vi "OSC_Calc-1.vi"(8 "Flow":dbl, 9 "Lambda 2 Array":dbl[](array[numeric]), 10 "Lambda 1 Array":dbl[](array[numeric]), 11 "MFC":dbl) -> (1 "OSC-Meas Flow":dbl, 2 "OSC- Calc Flow":dbl, 3 "Calculated Flow":dbl)   [LabVIEW 2014]
uses:
  <vilib>/Analysis/baseanly.llb/Mean (DBL).vi
  <vilib>/Analysis/NI_AALPro.lvlib
  <vilib>/Analysis/NI_AALBase.lvlib
panel:
  out "After TP 1":i32
  out "After TP 2":i32
  out "Time":dbl
  out "mean":dbl format="%0.2f"
  out "mean 2":dbl format="%0.2f"
  out "mean 3":dbl format="%0.2f"
  out "L1 Gradient":dbl[](graph)
  out "L1 Avg Gradient":dbl[](graph)
  out "L1 Data":dbl[](graph)
  out "L1 Max Grad":dbl
  out "L1 TP":i32
  out "L2 Gradient":dbl[](graph)
  out "L2 Avg Gradient":dbl[](graph)
  out "L2 Data":dbl[](graph)
  out "L2 Max Grad":dbl
  out "L2 TP":i32
  # "OSC Calculation"
  # "Inputs"
  # "Outputs"
  # "Indicators"
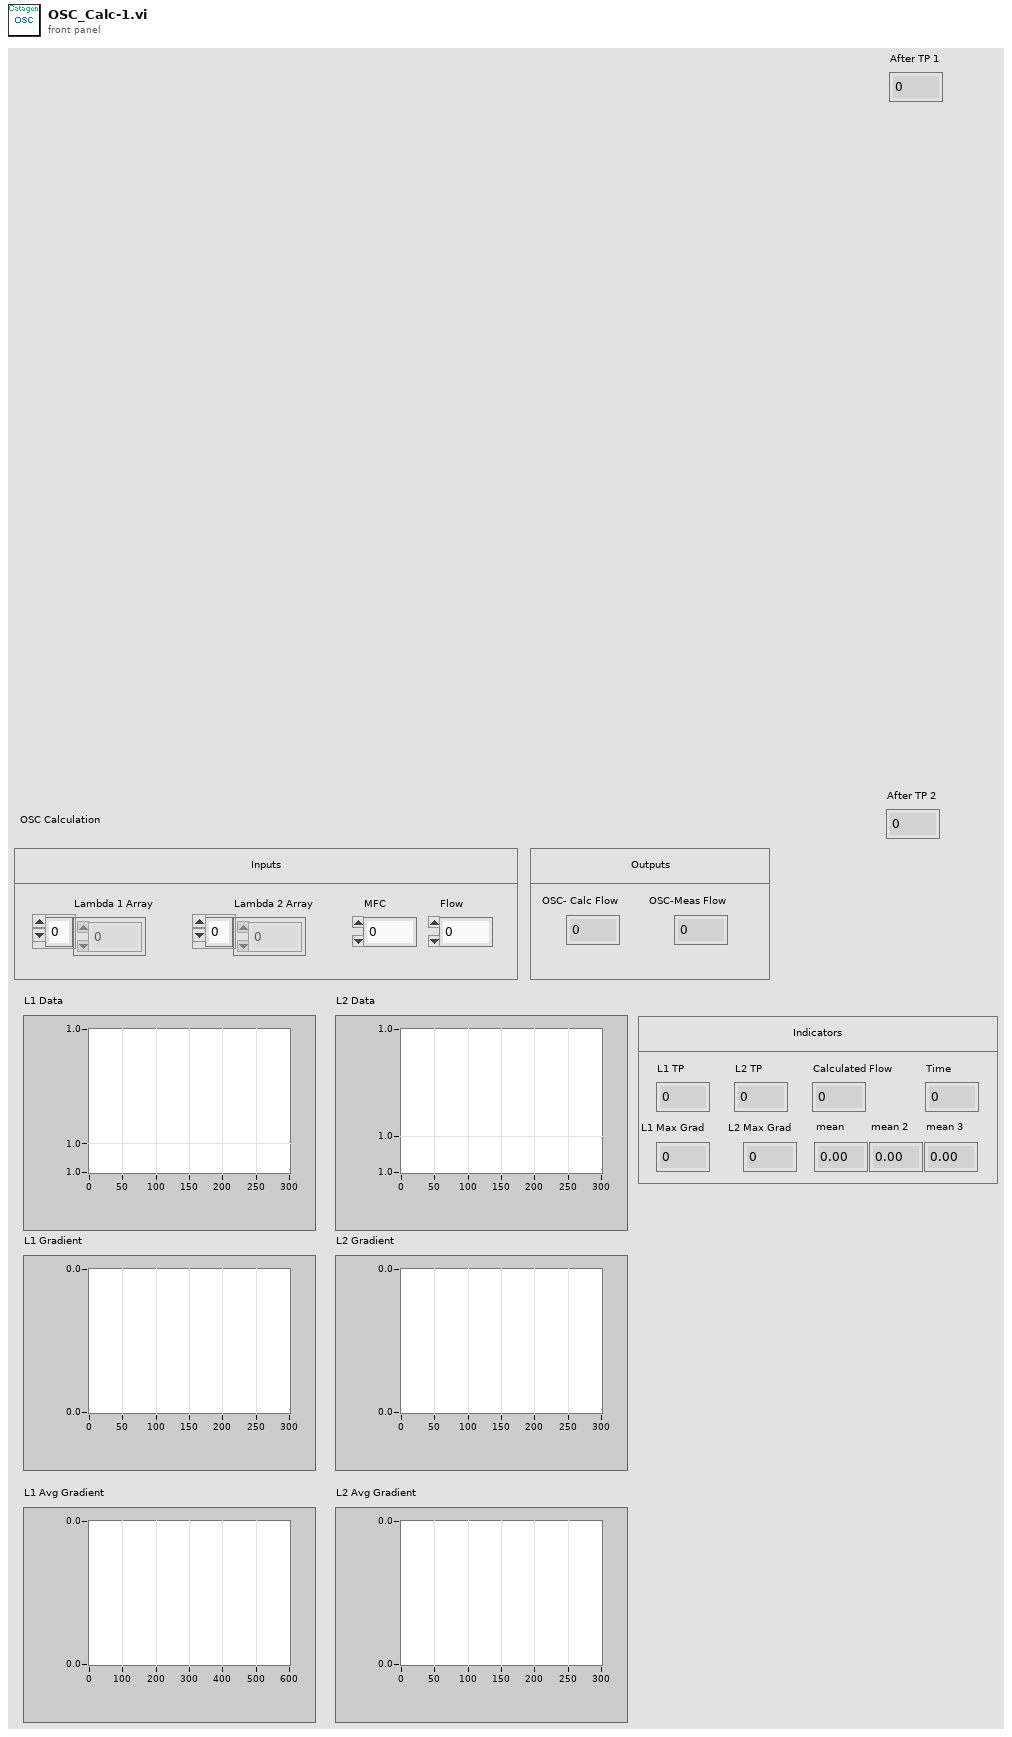
[diagram p1: front panel]
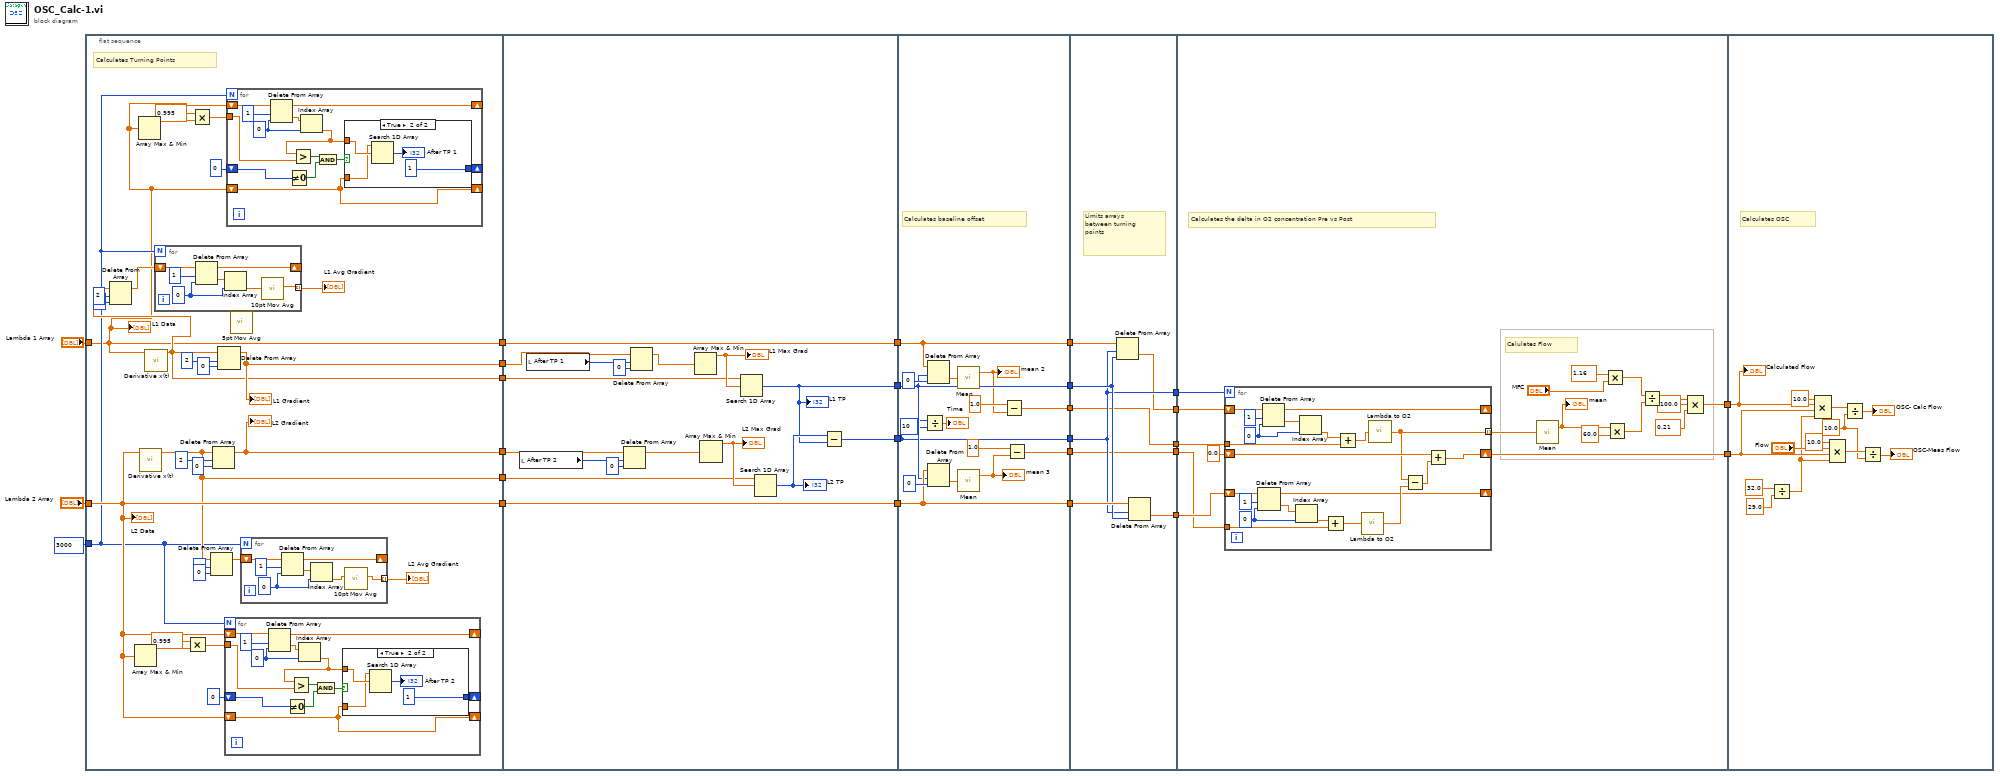
[diagram p0: block diagram]
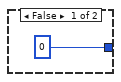
[diagram p2: hidden frame]
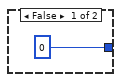
[diagram p3: hidden frame]
diagram:
  n1 = flat-sequence {
    tunnel: [w37] -> w10
    tunnel: [w27] -> w8
    tunnel: "Lambda 1 Array" -> [w27]
    tunnel: "Lambda 2 Array" -> [w37]
    tunnel: 3000 -> [w32]
    tunnel: [w36] -> w4
    tunnel: [w35] -> w3
    tunnel: [w34] -> w2
    tunnel: [w33] -> w1
    tunnel: w10 -> [w120]
    tunnel: [w120] -> w9
    tunnel: w8 -> [w119]
    tunnel: [w119] -> w7
    tunnel: [w115] -> w6
    tunnel: [w104] -> w5
    tunnel: w4 -> [w105]
    tunnel: w3 -> [w114]
    tunnel: w2 -> [w113]
    tunnel: w1 -> [w112]
    tunnel: w9 -> [w131]
    tunnel: [w131] -> w26
    tunnel: w7 -> [w136]
    tunnel: [w136] -> w25
    tunnel: w6 -> [w123]
    tunnel: [w123] -> w24
    tunnel: w5 -> [w130]
    tunnel: [w130] -> w23
    tunnel: [w128] -> w22
    tunnel: [w124] -> w12
    tunnel: w26 -> [w143]
    tunnel: w25 -> [w144]
    tunnel: w24 -> [w141]
    tunnel: w23 -> [w142]
    tunnel: [w141] -> w21
    tunnel: [w140] -> w20
    tunnel: [w139] -> w19
    tunnel: w22 -> [w138]
    tunnel: [w138] -> w18
    tunnel: w12 -> [w137]
    tunnel: [w137] -> w11
    tunnel: w21 -> [w162]
    tunnel: w20 -> [w160]
    tunnel: w19 -> [w161]
    tunnel: [w158] -> w17
    tunnel: [w147] -> w16
    tunnel: w18 -> [w146]
    tunnel: w11 -> [w145]
    tunnel: w17 -> [w191]
    tunnel: w16 -> [w195]
    frame #0 {
      # "Calculates Turning Points"
      n2 = Array Max & Min(array=w37) -> (max value=w41:dbl)  [unwired: 3 out]
      n3 = Array Max & Min(array=w27) -> (max value=w30:dbl)  [unwired: 3 out]
      n4 = call <vilib>:"Derivative x(t).vi"("X"=w37) -> ("dX/dt"=w34:dbl[])  [unwired: 9 in, 1 out]
      n5 = call <vilib>:"Derivative x(t).vi"("X"=w27) -> ("dX/dt"=w35:dbl[])  [unwired: 9 in, 1 out]
      n6 = Delete From Array(array=w35, length=2, index=0) -> (array with subset deleted=w44:dbl[])  [unwired: 1 out]
      n7 = for {
        N: w32 -> [_]
        tunnel: [w97] -> w48 mode=indexing
        shift-right: [w102] -> _
        shift-left: w44 -> [w101]
        w99 = 0 ("index")
        n8 = Delete From Array(array=w101, length=1, index=w99) -> (deleted portion=w100:dbl[], array with subset deleted=w102:dbl[])
        n9 = Index Array(array=w100, index=w99) -> (element=w98:dbl)
        n10 = call "10pt Mov Avg.vi"("Value in"=w98) -> ("Value out"=w97:dbl)  [unwired: 10 in]
      }
      "L1 Avg Gradient" <- w48
      n11 = Multiply(x=0.995, y=w41) -> (x*y=w39:dbl)
      n12 = Multiply(x=0.995, y=w30) -> (x*y=w29:dbl)
      n13 = Delete From Array(array=w34, length=2, index=0) -> (array with subset deleted=w45:dbl[])  [unwired: 1 out]
      n14 = Delete From Array(array=w34, length=2, index=0) -> (array with subset deleted=w33:dbl[])  [unwired: 1 out]
      "L2 Gradient" <- w33
      n15 = Delete From Array(array=w35, length=2, index=0) -> (array with subset deleted=w36:dbl[])  [unwired: 1 out]
      "L1 Gradient" <- w36
      n16 = for {
        N: w32 -> [_]
        tunnel: w39 -> [w77]
        shift-right: [w84] -> _
        shift-left: w37 -> [w83]
        shift-right: [w74] -> _
        shift-left: 0 ("index") -> [w73]
        shift-right: [w72] -> _
        shift-left: w37 -> [w72]
        w81 = 0 ("index")
        n17 = Delete From Array(array=w83, length=1, index=w81) -> (deleted portion=w82:dbl[], array with subset deleted=w84:dbl[])
        n18 = Not Equal To 0?(x=w73) -> (x != 0?=w75:bool)
        n19 = Index Array(array=w82, index=w81) -> (element=w76:dbl)
        n20 = Greater?(x=w76, y=w77) -> (0:w78:bool)
        n21 = And(x=w78, y=w75) -> (x .and. y?=w79:bool)
        n22 = case shown="True" w79 {
          tunnel: w76 -> [_ w88]
          tunnel: [0 ("index") 1 ("index")] -> w74
          tunnel: w72 -> [_ w87]
          frame False {
          }
          frame True {
            n23 = Search 1D Array(1D array=w87, element=w88) -> (index of element=→"After TP 2":i32)  [unwired: 1 in]
          }
        }
      }
      n24 = for {
        N: w32 -> [_]
        tunnel: w29 -> [w59]
        shift-right: [w66] -> _
        shift-left: w27 -> [w65]
        shift-right: [w56] -> _
        shift-left: 0 ("index") -> [w55]
        shift-right: [w54] -> _
        shift-left: w27 -> [w54]
        w63 = 0 ("index")
        n25 = Delete From Array(array=w65, length=1, index=w63) -> (deleted portion=w64:dbl[], array with subset deleted=w66:dbl[])
        n26 = Not Equal To 0?(x=w55) -> (x != 0?=w57:bool)
        n27 = Index Array(array=w64, index=w63) -> (element=w58:dbl)
        n28 = Greater?(x=w58, y=w59) -> (0:w60:bool)
        n29 = And(x=w60, y=w57) -> (x .and. y?=w61:bool)
        n30 = case shown="True" w61 {
          tunnel: w58 -> [_ w70]
          tunnel: [0 ("index") 1 ("index")] -> w56
          tunnel: w54 -> [_ w69]
          frame False {
          }
          frame True {
            n31 = Search 1D Array(1D array=w69, element=w70) -> (index of element=→"After TP 1":i32)  [unwired: 1 in]
          }
        }
      }
      n32 = call "5pt Mov Avg.vi"() -> ()  [unwired: 11 in, 1 out]
      n33 = for {
        N: w32 -> [_]
        tunnel: [w90] -> w49 mode=indexing
        shift-right: [w95] -> _
        shift-left: w45 -> [w94]
        w92 = 0 ("index")
        n34 = Delete From Array(array=w94, length=1, index=w92) -> (deleted portion=w93:dbl[], array with subset deleted=w95:dbl[])
        n35 = Index Array(array=w93, index=w92) -> (element=w91:dbl)
        n36 = call "10pt Mov Avg.vi"("Value in"=w91) -> ("Value out"=w90:dbl)  [unwired: 10 in]
      }
      "L2 Avg Gradient" <- w49
      "L1 Data" <- w27
      "L2 Data" <- w37
    }
    frame #1 {
      n37 = local read "After TP 2"() -> (w109:i32)
      n38 = local read "After TP 1"() -> (w108:i32)
      n39 = Delete From Array(array=w112, length=w109, index=0) -> (array with subset deleted=w111:dbl[])  [unwired: 1 out]
      n40 = Delete From Array(array=w105, length=w108, index=0) -> (array with subset deleted=w106:dbl[])  [unwired: 1 out]
      n41 = Array Max & Min(array=w106) -> (max value=w116:dbl)  [unwired: 3 out]
      "L1 Max Grad" <- w116
      n42 = Array Max & Min(array=w111) -> (max value=w117:dbl)  [unwired: 3 out]
      "L2 Max Grad" <- w117
      n43 = Search 1D Array(1D array=w114, element=w116) -> (index of element=w104:i32)  [unwired: 1 in]
      "L1 TP" <- w104
      n44 = Search 1D Array(1D array=w113, element=w117) -> (index of element=w118:i32)  [unwired: 1 in]
      "L2 TP" <- w118
      n45 = Subtract(x=w118, y=w104) -> (x-y=w115:i32)
    }
    frame #2 {
      # "Calculates baseline offset"
      n46 = Divide(x=w123, y=10) -> (x/y=→"Time":dbl)
      n47 = Delete From Array(array=w136, length=w130, index=0) -> (deleted portion=w134:dbl[])  [unwired: 1 out]
      n48 = Delete From Array(array=w131, length=w130, index=0) -> (deleted portion=w133:dbl[])  [unwired: 1 out]
      n49 = call-poly <vilib>:"Mean.vi"("X"=w134) -> ("mean"=w126:dbl)  [unwired: 1 out]
      "mean 2" <- w126
      n50 = call-poly <vilib>:"Mean.vi"("X"=w133) -> ("mean"=w129:dbl)  [unwired: 1 out]
      "mean 3" <- w129
      n51 = Subtract(x=1.0, y=w126) -> (x-y=w124:dbl)
      n52 = Subtract(x=1.0, y=w129) -> (x-y=w128:dbl)
    }
    frame #3 {
      # "Limits arrays\nbetween turning\npoints"
      n53 = Delete From Array(array=w144, length=w141, index=w142) -> (deleted portion=w139:dbl[])  [unwired: 1 out]
      n54 = Delete From Array(array=w143, length=w141, index=w142) -> (deleted portion=w140:dbl[])  [unwired: 1 out]
    }
    frame #4 {
      # "Calculates the delta in O2 concentration Pre vs Post"
      # "Calulates Flow"
      n55 = for {
        N: w162 -> [_]
        shift-right: [w170] -> _
        shift-left: w161 -> [w183]
        shift-right: [w169] -> _
        shift-left: w160 -> [w176]
        shift-right: [w174] -> w158
        shift-left: 0.0 ("element") -> [w175]
        tunnel: [w171] -> w157 mode=indexing
        tunnel: w146 -> [w167]
        tunnel: w145 -> [w164]
        w179 = 0 ("index")
        w180 = 0 ("index")
        n56 = Delete From Array(array=w176, length=1, index=w179) -> (deleted portion=w178:dbl[], array with subset deleted=w169:dbl[])
        n57 = Delete From Array(array=w183, length=1, index=w180) -> (deleted portion=w181:dbl[], array with subset deleted=w170:dbl[])
        n58 = Index Array(array=w178, index=w179) -> (element=w168:dbl)
        n59 = Index Array(array=w181, index=w180) -> (element=w165:dbl)
        n60 = Add(x=w168, y=w167) -> (x+y=w166:dbl)
        n61 = Add(x=w165, y=w164) -> (x+y=w163:dbl)
        n62 = call "Lambda to O2.vi"("Lambda"=w166) -> ("O2 %"=w172:sgl)
        n63 = call "Lambda to O2.vi"("Lambda"=w163) -> ("O2 %"=w171:sgl)
        n64 = Subtract(x=w171, y=w172) -> (x-y=w173:sgl)
        n65 = Add(x=w175, y=w173) -> (x+y=w174:dbl)
      }
      n66 = call-poly <vilib>:"Mean.vi"("X"=w157) -> ("mean"=w154:dbl)  [unwired: 1 out]
      "mean" <- w154
      n67 = Multiply(x=1.16, y="MFC") -> (x*y=w152:dbl)
      n68 = Multiply(x=w154, y=60.0) -> (x*y=w151:dbl)
      n69 = Divide(x=w152, y=w151) -> (x/y=w150:dbl)
      n70 = Compound Arithmetic op=MULTIPLY(w150, 100.0 ("value"), 0.21 ("value")) -> (w147:dbl)
    }
    frame #5 {
      w184 = 10.0 ("y")
      # "Calculates OSC"
      n71 = Divide(x=32.0, y=29.0) -> (x/y=w189:dbl)
      n72 = Compound Arithmetic op=MULTIPLY(10.0 ("value"), w195, w191, w189) -> (w185:dbl)
      n73 = Compound Arithmetic op=MULTIPLY(10.0 ("value"), "Flow", w191, w189) -> (w186:dbl)
      n74 = Divide(x=w185, y=w184) -> (x/y=→"OSC- Calc Flow":dbl)
      n75 = Divide(x=w186, y=w184) -> (x/y=→"OSC-Meas Flow":dbl)
      "Calculated Flow" <- w195
    }
  }
